vi "Gyro Tasks.vi"   [LabVIEW 2017]
uses:
  Implementation/Drive Published Globals.vi
  ADIS16448 IMU/ADIS16448_IMU.lvlib
types:
  T1 = typedef "ADIS16448_IMU.lvlib/ADI_IMU_ADIS16448_IMUDevRef.ctl" = cluster{"DevStatus":errorcluster, "Handle":i32, "SPI Bus":T2, "Device Found":bool, "Device Ready":bool, "Yaw Axis":enum16{"X", "Y", "Z"}, "AHRS Algorithm":enum16{"Complementary", "Madgwick"}, "Serial":u16, "Lot ID 2":u16, "Lot ID 1":u16, "Bytes Per Sample":u16, "Calibrate On Open?":bool}
  T2 = typedef "spi_bus.ctl" = enum16{"SPI On-Board, CS0", "SPI On-Board, CS1", "SPI On-Board, CS2", "SPI On-Board, CS3", "SPI MXP", "Invalid"}
  T3 = cluster{"X Angle":dbl, "Y Angle":dbl, "Z Angle":dbl}
  T4 = cluster{"X Gyro":dbl, "Y Gyro":dbl, "Z Gyro":dbl, "X Accel":dbl, "Y Accel":dbl, "Z Accel":dbl, "X Mag":dbl, "Y Mag":dbl, "Z Mag":dbl, "Pressure":dbl, "Temp":dbl}
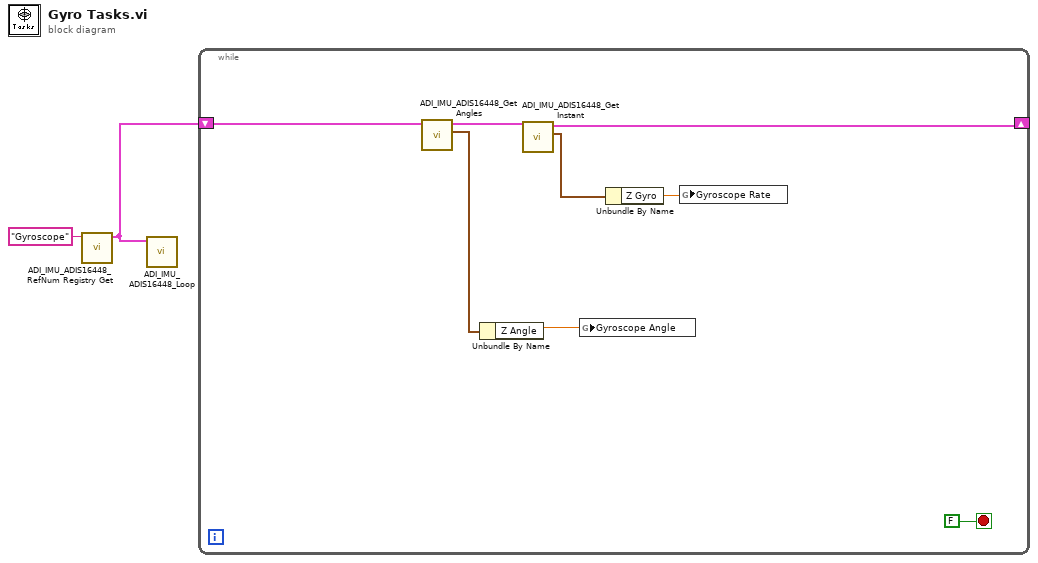
[diagram p0: block diagram]
diagram:
  n1 = call "ADI_IMU_ADIS16448_RefNum Registry Get.vi"("refnum name"="Gyroscope") -> ("ADI IMU DevRef"=w1:T1)  [unwired: 9 in, 1 out]
  n2 = call "ADI_IMU_ADIS16448_Loop.vi"("ADI IMU DevRef"=w1) -> ()  [unwired: 10 in, 1 out]
  n3 = while {
    shift-right: [w4] -> _
    shift-left: w1 -> [w8]
    stop <- FALSE stop-if-true
    n4 = call "ADI_IMU_ADIS16448_Get Angles.vi"("ADI IMU DevRef"=w8) -> ("IMU Angles Out"=w10:T3, "ADI IMU DevRef Out"=w5:T1)  [unwired: 7 in, 2 out]
    n5 = Unbundle By Name(w10) -> ("Z Angle"=w7:dbl)
    n6 = call "ADI_IMU_ADIS16448_Get Instant.vi"("ADI IMU DevRef"=w5) -> ("IMU Data Out"=w6:T4, "ADI IMU DevRef Out"=w4:T1)  [unwired: 7 in, 2 out]
    n7 = global write "Drive Published Globals.vi" "Gyroscope Angle"(w7) -> ()
    n8 = Unbundle By Name(w6) -> ("Z Gyro"=w3:dbl)
    n9 = global write "Drive Published Globals.vi" "Gyroscope Rate"(w3) -> ()
  }
